vi "设定压力.vi"(2 "error in (no error) 2":errorcluster caption="错误输入（无错误）", 3 "设定":dbl, 4 "VISA resource name":refnum<visa-resource-name> caption="VISA资源名称") -> (0 "错误输出":errorcluster, 1 "VISA资源名称输出":refnum<visa-resource-name>)   [LabVIEW 2017]
panel:
  out "设定压力值":string
  in  "等待时间（毫秒）":u32=100
  in  "写":bool=TRUE
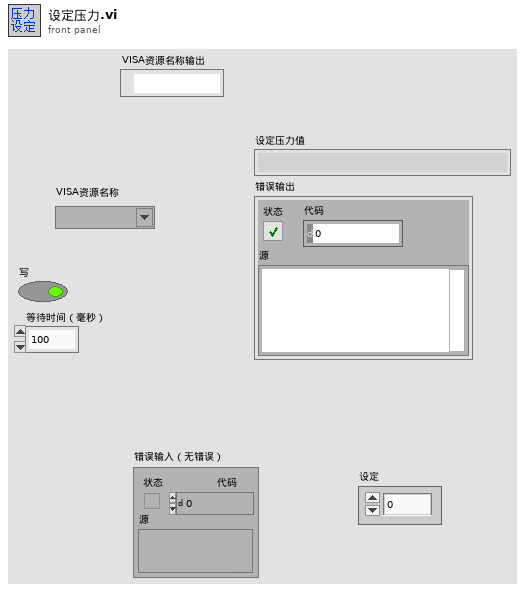
[diagram p1: front panel]
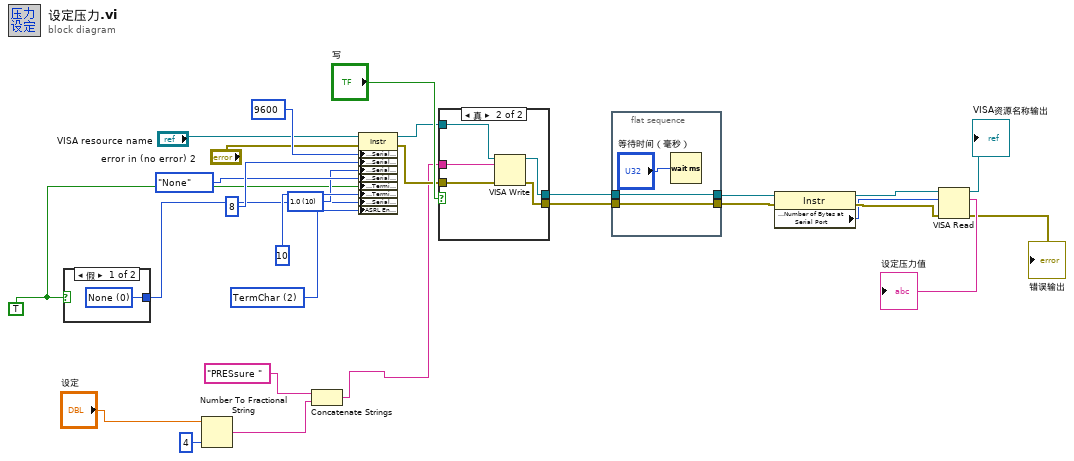
[diagram p0: block diagram]
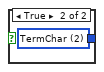
[diagram p2: hidden frame]
diagram:
  w11 = TRUE ("Enable Termination\nChar (T) 2")
  w10 = u16 2 items=["None", "Last Bit", "TermChar", "Break"] ("Serial Settings:End Mode for Writes")
  w13 = u16 10 items=["1.0"=10, "1.5"=15, "2.0"=20] ("stop bits (10: 1 bit)")
  n1 = case shown="假" w11 {
    tunnel: [w29 w30] -> w12
    frame False {
      w29 = u16 0 items=["None", "LastBit", "TermChar"] ("Serial Settings:Serial End Mode for Reads")
    }
    frame True {
      w30 = u16 2 items=["None", "LastBit", "TermChar"] ("Serial Settings:Serial End Mode for Reads")
    }
  }
  n2 = Number To Fractional String(number="设定", precision (6)=i16 4 ("精度(6)")) -> (F-format string=w3:string)  [unwired: 2 in]
  n3 = Concatenate Strings("PRESsure ", w3) -> (w1:string)
  n4 = property class="Instr"(reference="VISA resource name", error in="error in (no error) 2", "Serial Settings:Serial Baud Rate"=u32 9600 ("baud rate (9600)"), "Serial Settings:Serial Data Bits"=u16 8 ("data bits (8)"), "Serial Settings:Serial Stop Bits"=w13, "Serial Settings:Serial Parity"=enum16{"None", "Odd", "Even", "Mark", "Space"}."None" ("parity (0:none)"), "Message Based Settings:Termination Character Enable"=w11, "Message Based Settings:Termination Character"=u8 10 ("termination char\n(0xA = '\\n' = LF)"), "Serial Settings:Serial End Mode for Reads"=w12, "ASRL End Out"=w10) -> (reference out=w9:refnum<visa-resource-name>, error out=w8:errorcluster)
  n5 = case shown="真" "写" {
    tunnel: w1 -> [_ w37]
    tunnel: [w32 w36] -> w27
    tunnel: [w31 w35] -> w26
    tunnel: w9 -> [w31 w34]
    tunnel: w8 -> [w32 w33]
    frame False {
    }
    frame True {
      n6 = VISA Write(VISA resource name=w34, write buffer=w37, error in (no error)=w33) -> (VISA resource name out=w35:refnum<visa-resource-name>, error out=w36:errorcluster)  [unwired: 1 out]
    }
  }
  n7 = flat-sequence {
    tunnel: w27 -> [w38]
    tunnel: w26 -> [w39]
    tunnel: [w39] -> w23
    tunnel: [w38] -> w22
    frame #0 {
      n8 = Wait (ms)(milliseconds to wait="等待时间（毫秒）") -> ()  [unwired: 1 out]
    }
  }
  n9 = property class="Instr"(reference=w23, error in=w22) -> (reference out=w25:refnum<visa-resource-name>, error out=w24:errorcluster, "Serial Settings:Number of Bytes at Serial Port"=w21:u32)
  n10 = VISA Read(VISA resource name=w25, byte count=w21, error in (no error)=w24) -> (VISA resource name out=→"VISA资源名称输出":refnum<visa-resource-name>, read buffer=→"设定压力值":string, error out=→"错误输出":errorcluster)  [unwired: 1 out]
